vi "UnmaskPayload.vi"(5 "mask value":u32 format="%.0x", 8 "payload":string) -> (2 "unmasked payload":string)   [LabVIEW 2014, in "Raspberry Pi Compatible Compiler for LabVIEW.lvlib" / "Websocket.lvlib"]
uses:
  Websocket.lvlib
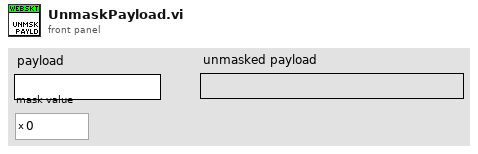
[diagram p1: front panel]
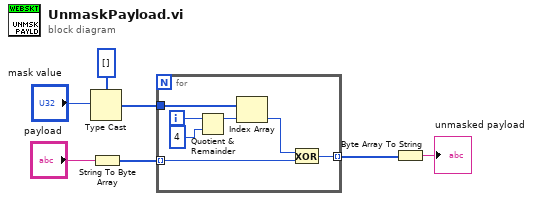
[diagram p0: block diagram]
diagram:
  n1 = Type Cast(type=u8[] [], x="mask value") -> (*(type *) &x=w2:u8[])
  n2 = String To Byte Array(string="payload") -> (unsigned byte array=w4:u8[])
  n3 = for {
    tunnel: w2 -> [w14]
    tunnel: w4 -> [w10] mode=indexing
    tunnel: [w8] -> w1 mode=indexing
    i -> [w12]
    n4 = Quotient & Remainder(x=w12, y=4) -> (x-y*floor(x/y)=w13:i32)  [unwired: 1 out]
    n5 = Index Array(array=w14, index=w13) -> (element=w9:u8)
    n6 = Exclusive Or(1:w10, 2:w9) -> (0:w8:u8)
  }
  n7 = Byte Array To String(unsigned byte array=w1) -> (string=→"unmasked payload":string)
